vi "Read Control Parameters.vi"(8 "error in (no error)":errorcluster, 11 "Lakeshore 325 in":refnum<class "Lakeshore 325.lvclass">) -> (0 "error out":errorcluster, 2 "Control Parameters":cluster{"P":dbl, "I":dbl, "D":u16}[](array[cluster]), 3 "Lakeshore 325 out":refnum<class "Lakeshore 325.lvclass">)   [LabVIEW 2022 SP3, in "Lakeshore 325.lvclass"]
uses:
  Lakeshore 325.lvclass
  Lakeshore 325.lvclass/Lakeshore 325.ctl
  Temp Control.lvclass
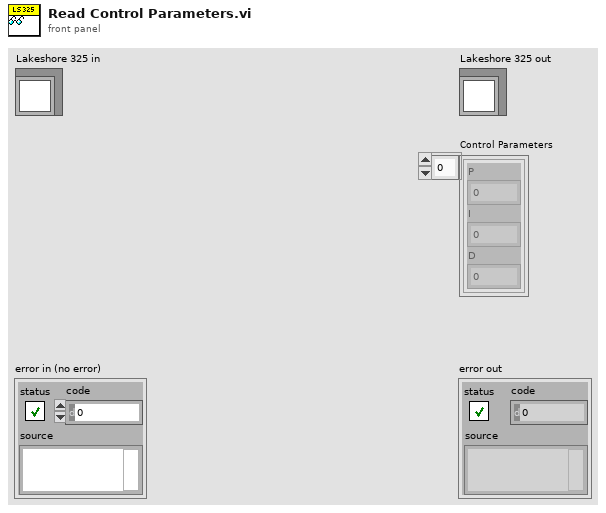
[diagram p1: front panel]
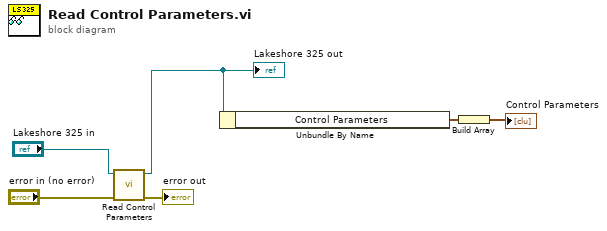
[diagram p0: block diagram]
diagram:
  n1 = call-parent "Read Control Parameters.vi"("error in (no error)"="error in (no error)", "Temp Control in"="Lakeshore 325 in") -> ("error out"=→"error out":errorcluster, "Temp Control out"=w3:refnum<class "Lakeshore 325.lvclass">)  [unwired: 7 in, 1 out]
  "Lakeshore 325 out" <- w3
  n2 = Unbundle By Name(w3) -> ("Control Parameters"=w2:cluster{"P":dbl, "I":dbl, "D":u16})
  n3 = Build Array(w2) -> (→"Control Parameters":cluster{"P":dbl, "I":dbl, "D":u16}[])
